vi "TestLINX.vi"() -> ()   [LabVIEW 2014]
uses:
  <vilib>/Instr/_visa.llb/VISA Find Search Mode.ctl
panel:
  out "4000":bool
  out "2000":bool
  out "1000":bool
  out "500":bool
  out "find list":string[](array[string])
  in  "stop":bool
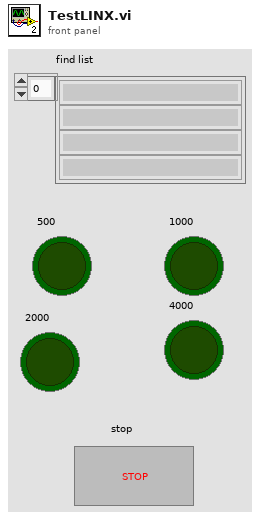
[diagram p1: front panel]
types:
  T1 = typedef "VISA Find Search Mode.ctl" = u32
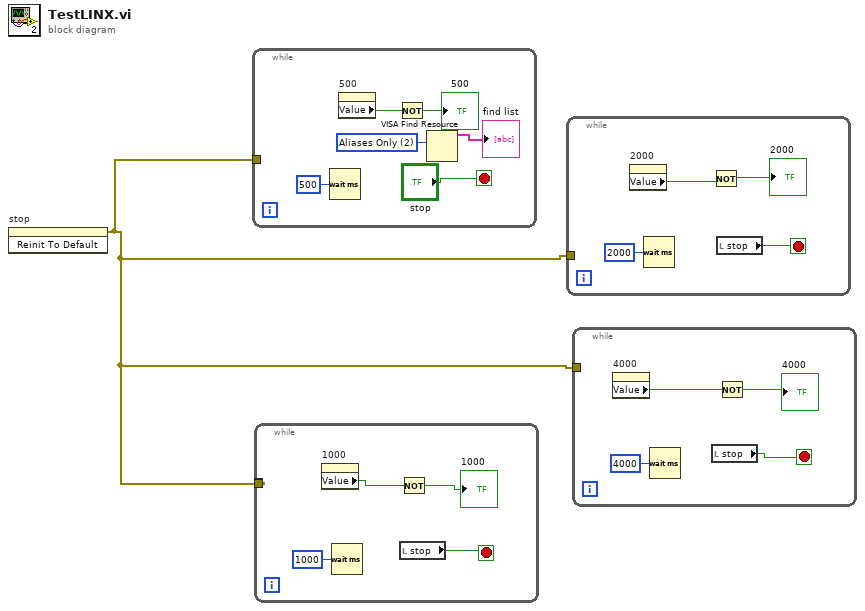
[diagram p0: block diagram]
diagram:
  n1 = invoke on="stop" class="Bool (strict)" method="Reinit To Default"() -> (error out=w1:errorcluster)  [unwired: 3 in, 2 out]
  n2 = while {
    tunnel: w1 -> [_]
    stop <- "stop" stop-if-true
    w3 = T1 2 items=["Canonical Names Only"=0, "Aliases Only"=2, "Include Matching Aliases"=3, "Include All Aliases"=4] ("Search Mode")
    n3 = Wait (ms)(milliseconds to wait=u32 500) -> ()  [unwired: 1 out]
    n4 = property on="500" class="Bool (strict)"() -> ("Value"=w5:bool)  [unwired: 2 in, 2 out]
    n5 = Not(x=w5) -> (.not. x?=→"500":bool)
    n6 = VISA Find Resource(10:w3) -> (3:→"find list":string[])  [unwired: 2 in, 2 out]
  }
  n7 = while {
    tunnel: [w8] -> _
    tunnel: w1 -> [w8]
    stop <- w9 stop-if-true
    n8 = property on="1000" class="Bool (strict)"() -> ("Value"=w10:bool)  [unwired: 2 in, 2 out]
    n9 = Wait (ms)(milliseconds to wait=u32 1000) -> ()  [unwired: 1 out]
    n10 = Not(x=w10) -> (.not. x?=→"1000":bool)
    n11 = local read "stop"() -> (w9:bool)
  }
  n12 = while {
    tunnel: w1 -> [_]
    stop <- w13 stop-if-true
    n13 = property on="2000" class="Bool (strict)"() -> ("Value"=w14:bool)  [unwired: 2 in, 2 out]
    n14 = Wait (ms)(milliseconds to wait=u32 2000) -> ()  [unwired: 1 out]
    n15 = Not(x=w14) -> (.not. x?=→"2000":bool)
    n16 = local read "stop"() -> (w13:bool)
  }
  n17 = while {
    tunnel: w1 -> [_]
    stop <- w17 stop-if-true
    n18 = property on="4000" class="Bool (strict)"() -> ("Value"=w18:bool)  [unwired: 2 in, 2 out]
    n19 = Wait (ms)(milliseconds to wait=u32 4000) -> ()  [unwired: 1 out]
    n20 = local read "stop"() -> (w17:bool)
    n21 = Not(x=w18) -> (.not. x?=→"4000":bool)
  }
